vi "Autonomous Indictactor.vi"(11 "Int In":dbl) -> (3 "String Out":string)   [LabVIEW 2014]
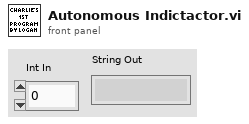
[diagram p1: front panel]
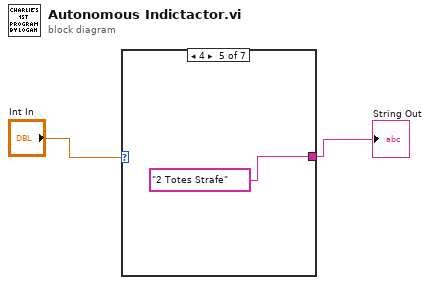
[diagram p0: block diagram]
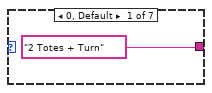
[diagram p2: hidden frame]
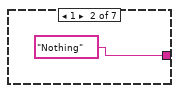
[diagram p3: hidden frame]
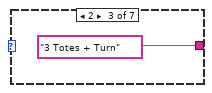
[diagram p4: hidden frame]
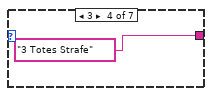
[diagram p5: hidden frame]
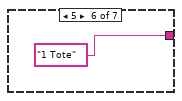
[diagram p6: hidden frame]
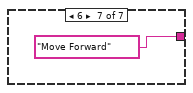
[diagram p7: hidden frame]
diagram:
  n1 = case shown="4" "Int In" {
    tunnel: ["2 Totes + Turn" "Nothing" "3 Totes + Turn" "3 Totes Strafe" "2 Totes Strafe" "1 Tote" "Move Forward"] -> w1
    frame 0, Default {
    }
    frame 1 {
    }
    frame 2 {
    }
    frame 3 {
    }
    frame 4 {
    }
    frame 5 {
    }
    frame 6 {
    }
  }
  "String Out" <- w1
